vi "Acquire.vi"(6 "UI":refnum<queue>, 8 "error in (no error)":errorcluster, 9 "Data Queue":refnum<queue>, 10 "Data Notifier":refnum<notifier>, 11 "Hardware Resources in":T1) -> (0 "error out":errorcluster, 3 "Hardware Resources out":T1)   [LabVIEW 2014, in "AvaSpec.lvlib" / "AvaSpec Acquisition.lvlib"]
doc: "Perform the acquisition. Replace the contents of this diagram with calls to acquisition hardware."
uses:
  AvaSpec Acquisition.lvlib
  Hardware Configuration.ctl
  Libraries/AS-5216-DLL/AVS settings.ctl
  Sphere Indicator.ctl
  Settings/Measurement Type.ctl
  AvaSpec Color Parameters.ctl
  support/Message Queue/Message Cluster.ctl
  support/Message Queue/Enqueue Message (Single).vi
  support/Message Queue/AvaSpec Message Queue.lvlib
  AvaSpec.lvlib
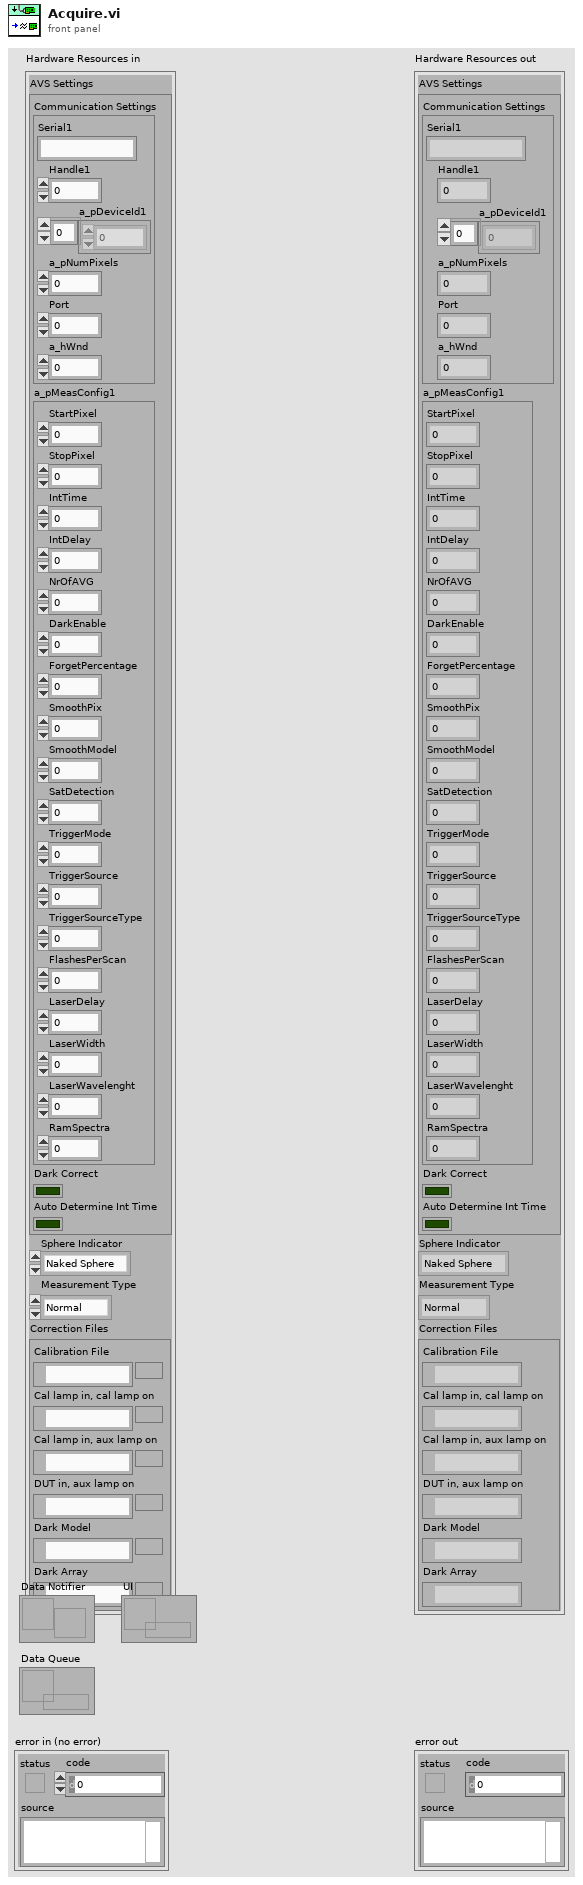
[diagram p1: front panel]
types:
  T1 = typedef "AvaSpec.lvlib/AvaSpec Acquisition.lvlib/Hardware Configuration.ctl" = cluster{"AVS Settings":T2, "Sphere Indicator":T3, "Measurement Type":T4, "Correction Files":cluster{"Calibration File":path, "Cal lamp in, cal lamp on":path, "Cal lamp in, aux lamp on":path, "DUT in, aux lamp on":path, "Dark Model":path, "Dark Array":path}}
  T2 = typedef "AvaSpec.lvlib/AVS settings.ctl" = cluster{"Communication Settings":cluster{"Serial1":string, "Handle1":i32, "a_pDeviceId1":u8[], "a_pNumPixels":u16, "Port":i32, "a_hWnd":i32}, "a_pMeasConfig1":cluster{"StartPixel":u16, "StopPixel":u16, "IntTime":sgl, "IntDelay":u32, "NrOfAVG":u32, "DarkEnable":u8, "ForgetPercentage":u8, "SmoothPix":u16, "SmoothModel":u8, "SatDetection":u8, "TriggerMode":u8, "TriggerSource":u8, "TriggerSourceType":u8, "FlashesPerScan":u16, "LaserDelay":u32, "LaserWidth":u32, "LaserWavelenght":sgl, "RamSpectra":u16}, "Dark Correct":bool, "Auto Determine Int Time":bool}
  T3 = typedef "AvaSpec.lvlib/Sphere Indicator.ctl" = enum16{"Naked Sphere", "Insulated Sphere"}
  T4 = typedef "AvaSpec.lvlib/AvaSpec Acquisition.lvlib/Measurement Type.ctl" = enum16{"Normal", "Calibration", "Dark"}
  T5 = typedef "AvaSpec.lvlib/AvaSpec Color Parameters.ctl" = cluster{"Power Spectral Distribution":cluster{"X":dbl, "Y":dbl}[], "Color Values":cluster{"luminousFlux":dbl, "CCT":dbl, "CRI":dbl, "u'":dbl, "v'":dbl, "Duv":dbl}, "R values":dbl[], "Chromaticity \nCoordinates":cluster{"x":dbl, "y":dbl, "z":dbl, "u":dbl, "v":dbl}, "Tristimulus \nValues":cluster{"X":dbl, "Y":dbl, "Z":dbl}, "Time Stamp":timestamp, "Temperature":dbl, "Integration Time":dbl, "Sphere Indicator":T3}
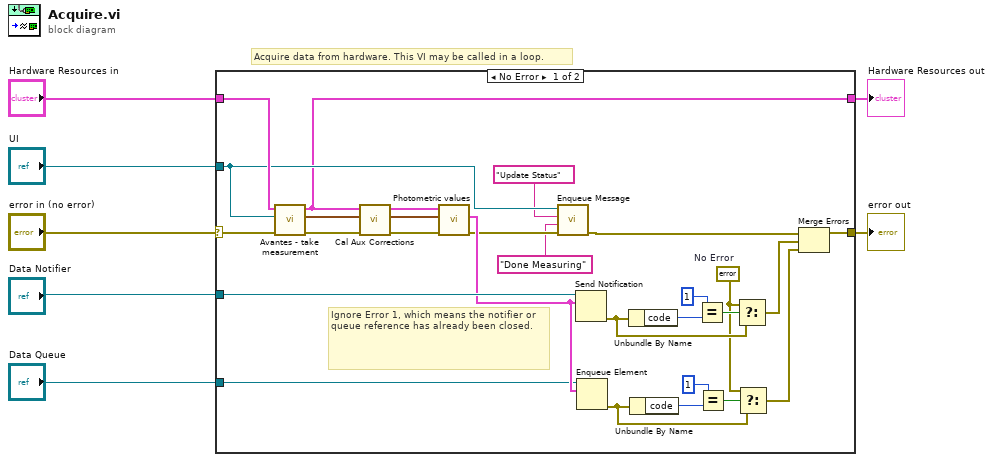
[diagram p0: block diagram]
diagram:
  # "Acquire data from hardware. This VI may be called in a loop."
  n1 = case shown="No Error" "error in (no error)" {
    selector: "error in (no error)" -> [w22 w36]
    tunnel: [w35 w36] -> w6
    tunnel: "Hardware Resources in" -> [w21 w37]
    tunnel: [w13 w37] -> w4
    tunnel: "Data Notifier" -> [w34 _]
    tunnel: "Data Queue" -> [w19 _]
    tunnel: "UI" -> [w17 _]
    frame No Error {
      w23 = errorcluster {"status"=FALSE, "code"=0, "source"=""}  # No Error
      # "Ignore Error 1, which means the notifier or queue reference has already been closed."
      n2 = call "Avantes - take measurement.vi"("error in (no error)"=w22, "UI"=w17, "Hardware Resources in"=w21) -> ("error out"=w10:errorcluster, "Spectral distribution"=w14:cluster{dbl, dbl}[], "Hardware Resources out"=w13:T1)  [unwired: 6 in]
      n3 = call "Cal Aux Corrections.vi"("error in (no error)"=w10, "Spectral distribution In"=w14, "Hardware Resources in"=w13) -> ("error out"=w9:errorcluster, "Spectral distribution Out"=w11:cluster{dbl, dbl}[], "Hardware Resources out"=w12:T1)  [unwired: 6 in]
      n4 = call "Photometric values.vi"("error in (no error)"=w9, "Power Spectral Distribution"=w11, "Hardware Resources in"=w12) -> ("error out"=w18:errorcluster, "Color Parameters out"=w20:T5)  [unwired: 7 in]
      n5 = call-poly "Enqueue Message.vi"("error in (no error)"=w18, "Message Data"="Done Measuring" ("Message"), "Message"="Update Status", "Message Queue"=w17) -> ("error out"=w8:errorcluster)  [unwired: 6 in, 1 out]
      n6 = Send Notification(notification=w20, notifier=w34) -> (error out=w30:errorcluster)  [unwired: 1 in, 1 out]
      n7 = Enqueue Element(queue=w19, element=w20) -> (error out=w28:errorcluster)  [unwired: 2 in, 2 out]
      n8 = Unbundle By Name(w30) -> ("code"=w33:i32)
      n9 = Unbundle By Name(w28) -> ("code"=w25:i32)
      n10 = Equal?(x=1, y=w33) -> (x = y?=w31:bool)
      n11 = Equal?(x=1, y=w25) -> (x = y?=w27:bool)
      n12 = Select(t=w23, s=w31, f=w30) -> (s? t:f=w29:errorcluster)
      n13 = Select(t=w23, s=w27, f=w28) -> (s? t:f=w24:errorcluster)
      n14 = Merge Errors(w8, w29, w24) -> (w35:errorcluster)
    }
    frame Error {
    }
  }
  "Hardware Resources out" <- w4
  "error out" <- w6
